vi "OAT Torsional Vibration (Analog Tacho) (Waveform) (N Ch - 1 Setting).vi"(0 "analog tacho signals":waveform(dbl)[](array[waveform]), 1 "threshold (auto)":dbl=inf, 2 "pulse/revolution (1)":i32=1 min=1, 3 "hysteresis (0)":dbl format="%.2g", 4 "torsional vibration units":enum16{"RPM", "deg/s", "rad/s"}(ring), 5 "error in (no error)":errorcluster, 6 "missing pulses? (no:F)":bool, 7 "pulse width (2)":i32=2 min=0, 8 "reset? (F)":bool, 9 "slope (Rising)":u16(ring) items=["Rising", "Falling"], 10 "compensate geometric imperfection? (F)":bool, 11 "output interval [s]":dbl=0.001 min=0.0) -> (14 "torsional vibration signals":waveform(dbl)[](array[waveform]), 15 "speed profiles":T1[](array[typedef]) {"speed [RPM]" format="%.2f"; "time [s]" format="%.2f"}, 18 "unit labels":string[](array[string]), 19 "error out":errorcluster)   [LabVIEW 2017, in "SoundVib_Torsional.lvlib"]
doc: "Calculates torsional vibration signals from analog tachometer signals. This VI can return torsional vibration signals as either waveform signals or even-angle signals. Wire data to the <B>analog tacho signal</B> input to determine the polymorphic instance to use or manually select the instance."
uses:
  <vilib>/addons/Sound and Vibration/Order Analysis/Torsional Vibration/SoundVib_Torsional.lvlib
  <vilib>/addons/Sound and Vibration/Order Analysis/Tach Process/SubVIs/speed profile.ctl
  <vilib>/addons/_NISVFA/_Shared subVIs/Common/svc_Check for Waveform Parameter Continuity (no state).vi
  <vilib>/addons/_NISVFA/_Shared subVIs/Common/svc_Get SV Channel Info.vi
  <vilib>/addons/_NISVFA/_Shared subVIs/Common/svc_Engineering Units to Unit Label.vi
  <vilib>/addons/_NISVFA/_Shared subVIs/Common/svc_Unit Label to Engineering Units.vi
  <vilib>/addons/Sound and Vibration/Order Analysis/Tach Process/SoundVib_TachProcess.lvlib
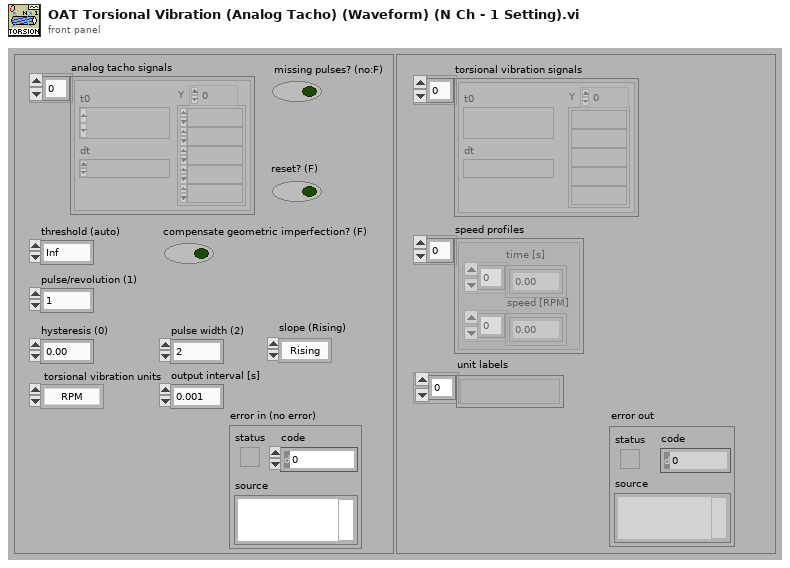
[diagram p1: front panel]
types:
  T1 = typedef "SoundVib_TachProcess.lvlib/speed profile.ctl" = cluster{"time [s]":dbl[], "speed [RPM]":dbl[]}
  T2 = cluster{"dt equal":bool, "array length equal":bool, "number channels change":bool}
  T3 = cluster{"dt":bool, "t0 continuity":bool, "array length":bool, "channel info":bool, "name":bool}
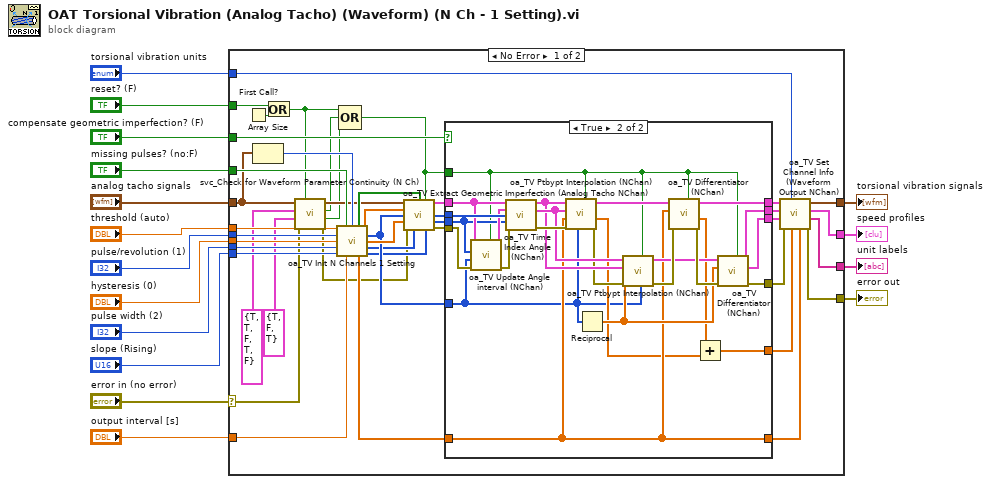
[diagram p0: block diagram]
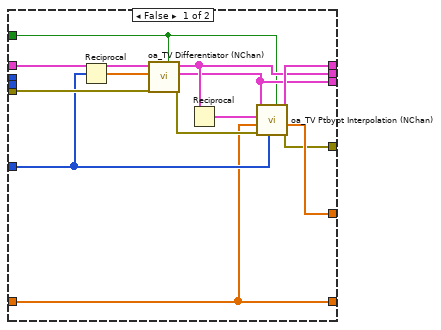
[diagram p2: hidden frame]
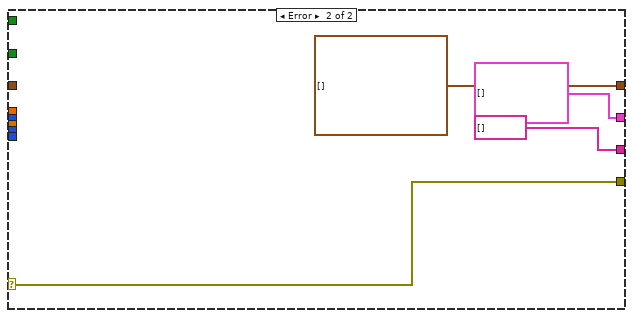
[diagram p3: hidden frame]
diagram:
  n1 = case shown="No Error" "error in (no error)" {
    selector: "error in (no error)" -> [w25 w101]
    tunnel: [w49 waveform(dbl)[] [] ("even time speed")] -> w12
    tunnel: [w50 w101] -> w16
    tunnel: "compensate geometric imperfection? (F)" -> [w43 _]
    tunnel: "reset? (F)" -> [w57 _]
    tunnel: "analog tacho signals" -> [w19 _]
    tunnel: "torsional vibration units" -> [w48 _]
    tunnel: [w46 T1[] [] ("speed profile")] -> w10
    tunnel: [w42 string[] [] ("unit labels")] -> w8
    tunnel: "threshold (auto)" -> [w39 _]
    tunnel: "pulse/revolution (1)" -> [w38 _]
    tunnel: "hysteresis (0)" -> [w37 _]
    tunnel: "output interval [s]" -> [w36 _]
    tunnel: "pulse width (2)" -> [w34 _]
    tunnel: "slope (Rising)" -> [w33 _]
    tunnel: "missing pulses? (no:F)" -> [w27 _]
    frame No Error {
      n2 = First Call?() -> (First Call?: T/F=w58:bool)
      n3 = Array Size(array=w19) -> (size(s)=w41:i32)
      n4 = Or(x=w57, y=w58) -> (x .or. y?=w23:bool)
      n5 = call <vilib>:"svc_Check for Waveform Parameter Continuity (N Ch).vi"("restart averaging (F)"=w23, "error in (no error)"=w25, "checks for multichannel parameters"=T2 {"dt equal"=TRUE, "array length equal"=FALSE, "number channels change"=TRUE}, "checks for channel parameter change"=T3 {"dt"=TRUE, "t0 continuity"=TRUE, "array length"=FALSE, "channel info"=TRUE, "name"=FALSE}, "scaled signal(s)"=w19) -> ("error out"=w24:errorcluster, "multichannel parameter changed"=w20:bool, "waveform parameter changed"=w21:bool, "dup scaled signal(s)"=w26:waveform(dbl)[])  [unwired: 3 out]
      n6 = call <vilib>:"oa_TV Init N Channels 1 Setting.vi"("threshold (auto)"=w39, "missing pulses? (no:F)"=w27, "channel number"=w41, "pulse/revolution (1)"=w38, "hysteresis (0)"=w37, "pulse width (2)"=w34, "slope (Rising)"=w33, "output interval [s]"=w36) -> ("missing pulses? out"=w40:bool[], "threshold out"=w32:dbl[], "pulse/revolution out"=w30:i32[], "hysteresis"=w31:dbl[], "pulse width out"=w29:i32[], "output interval"=w35:dbl[], "slope out"=w28:u16[])  [unwired: 1 in]
      n7 = Compound Arithmetic op=OR(w23, w21, w20) -> (w22:bool)
      n8 = call <vilib>:"oa_TV Extract Geometric Imperfection (Analog Tacho NChan).vi"("analog tacho signal"=w26, "missing pulses? (no:F)"=w40, "reset? (F)"=w22, "threshold (auto)"=w32, "pulse/revolution"=w30, "hysteresis(0)"=w31, "error in (no error)"=w24, "pulse width (2)"=w29, "slope (Rising)"=w28) -> ("pulse positions"=w54:cluster{dbl[]}[], "revulotion"=w56:i32[], "revulotion index"=w55:i32[], "error out"=w59:errorcluster)  [unwired: 3 in]
      n9 = case shown="True" w43 {
        tunnel: w59 -> [w70 w79]
        tunnel: w56 -> [_ w80]
        tunnel: w55 -> [_ w74]
        tunnel: w54 -> [w72 w76]
        tunnel: w30 -> [w67 w75]
        tunnel: [w63 w90] -> w53
        tunnel: [w62 w89] -> w52
        tunnel: [w64 w88] -> w51
        tunnel: w35 -> [w65 w84]
        tunnel: [w66 w82] -> w47
        tunnel: [w61 w85] -> w45
        tunnel: [w65 w84] -> w44
        tunnel: w22 -> [w60 w73]
        frame False {
          n10 = Reciprocal(x=w67) -> (1/x=w71:dbl[])
          n11 = call <vilib>:"oa_TV Differentiator (NChan).vi"("reset? (False)"=w60, "error in (no error)"=w70, "delta X"=w71, "Y[n]"=w72) -> ("error out"=w68:errorcluster, "X[n]"=w61:cluster{dbl[]}[], "dY[n]/dX[n]"=w62:cluster{dbl[]}[])  [unwired: 4 in, 1 out]
          n12 = Reciprocal(x=w62) -> (1/x=w69:cluster{dbl[]}[])
          n13 = call <vilib>:"oa_TV Ptbypt Interpolation (NChan).vi"("reset? (F)"=w60, "buffer size"=w67, "error in (no error)"=w68, "dX"=w65, "Y"=w69, "X"=w61) -> ("error out"=w64:errorcluster, "X0"=w66:dbl[], "resampled Y"=w63:cluster{dbl[]}[])  [unwired: 2 in, 1 out]
        }
        frame True {
          n14 = call <vilib>:"oa_TV Update Angle interval (NChan).vi"("reset? (F)"=w73, "error in (no error)"=w79, "pulse/revolution"=w75, "revulotion index"=w74, "pulse position [s]"=w76) -> ("error out"=w78:errorcluster, "angle intervals"=w77:cluster{dbl[]}[])  [unwired: 5 in]
          n15 = call <vilib>:"oa_TV Time Index Angle (NChan).vi"("pulse positions"=w76, "angle intervals"=w77, "revulotion"=w80, "revulotion index"=w74, "error in (no error)"=w78) -> ("pulse positions"=w94:cluster{dbl[]}[], "angle"=w95:cluster{dbl[]}[], "error out"=w97:errorcluster)  [unwired: 8 in]
          n16 = call <vilib>:"oa_TV Ptbypt Interpolation (NChan).vi"("reset? (F)"=w73, "buffer size"=w75, "error in (no error)"=w97, "dX"=w84, "Y"=w95, "X"=w94) -> ("error out"=w93:errorcluster, "X0"=w83:dbl[], "resampled Y"=w96:cluster{dbl[]}[])  [unwired: 2 in, 1 out]
          n17 = Reciprocal(x=w75) -> (1/x=w87:dbl[])
          n18 = call <vilib>:"oa_TV Ptbypt Interpolation (NChan).vi"("reset? (F)"=w73, "buffer size"=w75, "error in (no error)"=w93, "dX"=w87, "Y"=w94, "X"=w95) -> ("error out"=w92:errorcluster, "resampled Y"=w86:cluster{dbl[]}[])  [unwired: 2 in, 2 out]
          n19 = call <vilib>:"oa_TV Differentiator (NChan).vi"("reset? (False)"=w73, "error in (no error)"=w92, "delta X"=w84, "Y[n]"=w96) -> ("error out"=w91:errorcluster, "Delay"=w81:dbl[], "dY[n]/dX[n]"=w90:cluster{dbl[]}[])  [unwired: 4 in, 1 out]
          n20 = Add(x=w81, y=w83) -> (x+y=w82:dbl[])
          n21 = call <vilib>:"oa_TV Differentiator (NChan).vi"("reset? (False)"=w73, "error in (no error)"=w91, "delta X"=w87, "Y[n]"=w86) -> ("error out"=w88:errorcluster, "X[n]"=w85:cluster{dbl[]}[], "dY[n]/dX[n]"=w89:cluster{dbl[]}[])  [unwired: 4 in, 1 out]
        }
      }
      n22 = call <vilib>:"oa_TV Set Channel Info (Waveform Output NChan).vi"("dt"=w44, "t0"=w47, "torisional vibration unit (RPM)"=w48, "error in (no error)"=w51, "pulse position"=w45, "seconds/revolution"=w52, "revolutions/minute"=w53) -> ("error out"=w50:errorcluster, "unit labels"=w42:string[], "speed profile"=w46:T1[], "torsional vibration"=w49:waveform(dbl)[])  [unwired: 1 in]
    }
    frame Error {
    }
  }
  "error out" <- w16
  "torsional vibration signals" <- w12
  "speed profiles" <- w10
  "unit labels" <- w8
